vi "getMessage.vi"(8 "error in (no error)":errorcluster, 11 "AlCS in":refnum<class "AlCS.lvclass">) -> (0 "error out":errorcluster, 2 "message":string, 3 "AlCS out":refnum<class "AlCS.lvclass">)   [LabVIEW 2016, in "AlCS.lvclass"]
uses:
  AlCS.lvclass
  AlCS.lvclass/AlCS.ctl
  ts_labview_tcp/TCPClient/TCPClient.lvclass
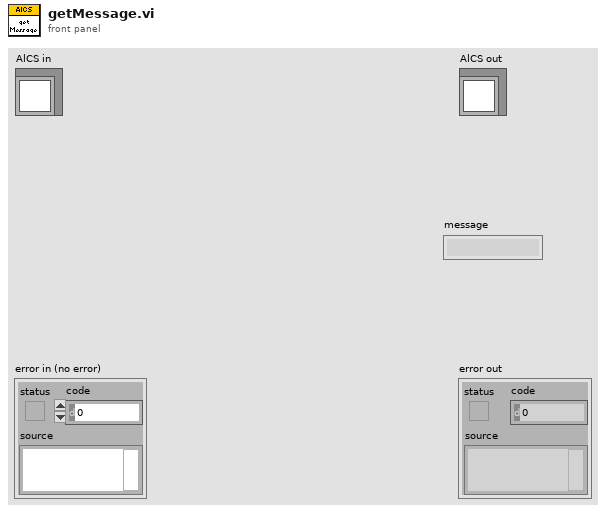
[diagram p1: front panel]
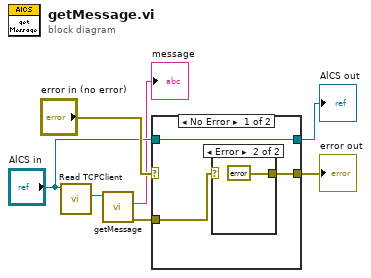
[diagram p0: block diagram]
diagram:
  n1 = call "Read TCPClient.vi"("AlCS in"="AlCS in") -> ("TCPClient.lvclass"=w3:refnum<class "TCPClient.lvclass">)  [unwired: 8 in, 2 out]
  n2 = call-dynamic "getMessage.vi"("TCPClient in"=w3) -> ("error out"=w1:errorcluster, "String"=→"message":string)  [unwired: 8 in, 1 out]
  n3 = case shown="No Error" "error in (no error)" {
    selector: "error in (no error)" -> [_ w14]
    tunnel: [w8 w14] -> w6
    tunnel: [w10 w13] -> w5
    tunnel: "AlCS in" -> [w10 w13]
    tunnel: w1 -> [w9 _]
    frame No Error {
      n4 = case shown="Error" w9 {
        selector: w9 -> [w11 _]
        tunnel: [w11 errorcluster {"status"=TRUE, "code"=8204, "source"="Monochromator Controller not responding"} ("error IO")] -> w8
        frame No Error {
        }
        frame Error {
        }
      }
    }
    frame Error {
    }
  }
  "error out" <- w6
  "AlCS out" <- w5
